vi "静态方法DEMO.vi"() -> ()   [LabVIEW 2013]
uses:
  Math.lvclass
panel:
  out "Root":dbl[](array[numeric])
  in  "ABC":dbl[](array[numeric])
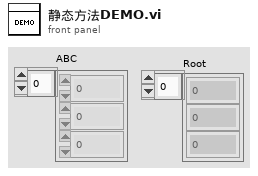
[diagram p1: front panel]
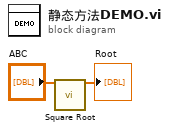
[diagram p0: block diagram]
diagram:
  n1 = call "Square Root.vi"("ABC"="ABC") -> ("Root"=→"Root":dbl[])  [unwired: 17 in, 1 out]
